vi "FileSaveTest.vi"() -> ()   [LabVIEW 2016]
uses:
  VIs/uPythonX/uPythonX.xctl
panel:
  out "Success?":bool
  out "Console Out":string
  in  "String":string
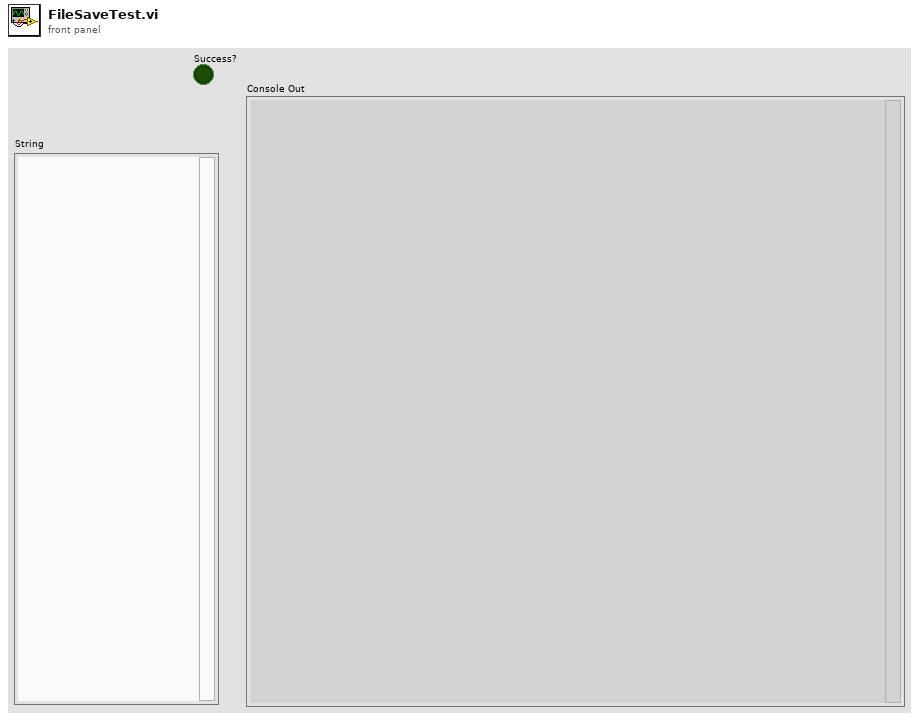
[diagram p1: front panel]
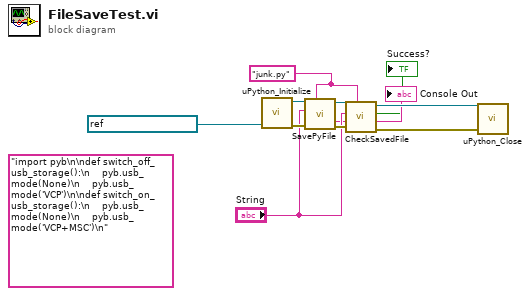
[diagram p0: block diagram]
diagram:
  (unwired) "import pyb\n\ndef switch_off_usb_storage():\n    pyb.usb_mode(None)\n    pyb.usb_mode('VCP')\n\ndef switch_on_usb_storage():\n    pyb.usb_mode(None)\n    pyb.usb_mode('VCP+MSC')\n" ("All Code")
  w8 = "junk.py" ("Name")
  n1 = call "uPython_Initialize.vi"("VISA Refnum in"=refnum<visa-resource-name> "ASRL44::INSTR") -> ("error out"=w11:errorcluster, "VISA Refnum out"=w12:refnum<visa-resource-name>)  [unwired: 9 in]
  n2 = call "SavePyFile.vi"("Name"=w8, "error in"=w11, "Python Code"="String", "VISA in"=w12) -> ("error out"=w10:errorcluster, "Reply"=w3:string, "VISA out"=w9:refnum<visa-resource-name>)  [unwired: 5 in]
  n3 = call "CheckSavedFile.vi"("Name"=w8, "error in (no error)"=w10, "Console in"=w3, "All Code"="String", "VISA in"=w9) -> ("error out"=w6:errorcluster, "Console Out"=→"Console Out":string, "Success?"=→"Success?":bool, "VISA out"=w7:refnum<visa-resource-name>)  [unwired: 3 in]
  n4 = call "uPython_Close.vi"("error in"=w6, "VISA  in"=w7) -> ()  [unwired: 8 in, 2 out]
